vi "Init Sync Stuff.vi"(8 "error in (no error)":errorcluster, 10 "DC Brick in":refnum<class "DC Brick.lvclass">) -> (0 "error out":errorcluster, 2 "DC Brick out":refnum<class "DC Brick.lvclass">)   [LabVIEW 2011, in "Tinkerforge.lvlib" / "DC Brick.lvclass"]
doc: "This VI is the child implementation of \"Init Sync Stuff.vi\" and initializes all synchronization objects of this child object."
uses:
  DC Brick.lvclass
  DC Brick.lvclass/DC Brick.ctl
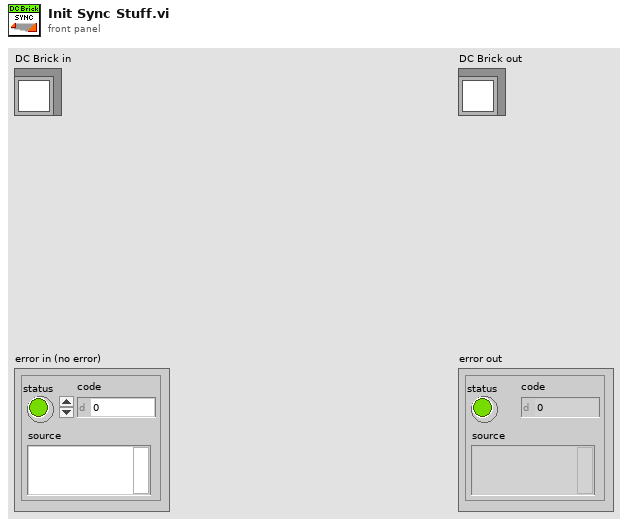
[diagram p1: front panel]
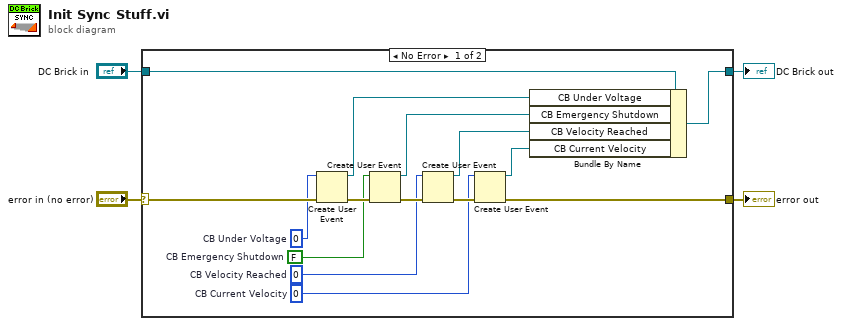
[diagram p0: block diagram]
diagram:
  n1 = case shown="No Error" "error in (no error)" {
    selector: "error in (no error)" -> [w17 w20]
    tunnel: "DC Brick in" -> [w19 w21]
    tunnel: [w9 w20] -> w2
    tunnel: [w18 w21] -> w1
    frame No Error {
      w10 = i16 0  # CB Current Velocity
      w12 = i16 0  # CB Velocity Reached
      w14 = FALSE  # CB Emergency Shutdown
      w16 = u16 0  # CB Under Voltage
      n2 = Create User Event(user event datatype=w16, error in=w17) -> (user event=w8:refnum<user-event>, error out=w15:errorcluster)
      n3 = Create User Event(user event datatype=w14, error in=w15) -> (user event=w7:refnum<user-event>, error out=w13:errorcluster)
      n4 = Create User Event(user event datatype=w12, error in=w13) -> (user event=w5:refnum<user-event>, error out=w11:errorcluster)
      n5 = Create User Event(user event datatype=w10, error in=w11) -> (user event=w6:refnum<user-event>, error out=w9:errorcluster)
      n6 = Bundle By Name(cluster=w19, "CB Under Voltage"=w8, "CB Emergency Shutdown"=w7, "CB Velocity Reached"=w5, "CB Current Velocity"=w6) -> (w18:refnum<class "DC Brick.lvclass">)
    }
    frame Error {
    }
  }
  "error out" <- w2
  "DC Brick out" <- w1
